vi "Autonomous Independent.vi"() -> ()   [LabVIEW 2016]
doc: "This VI is called when autonomous begins, and will automatically be terminated when autonomous ends. You can carry out timed or sensor driven robot movement independently without needing to return to the caller."
panel:
  out "ACTUAL Loop Time":u32
  # "Be sure to right-click and choose Data Operations>>Make Current Value default if you want to save the array values with the VI"
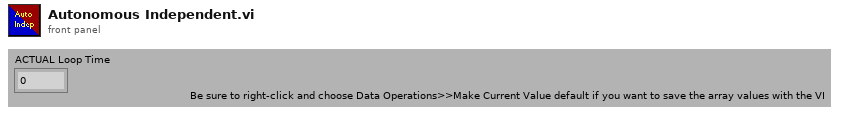
[diagram p1: front panel]
types:
  T1 = typedef "Autonomous Play Definition.ctl" = cluster{"Play Name":string, "Command List":cluster{"Param 1":dbl, "Param 2":dbl, "Autonomous Command Name":T2, "Concurrent":bool, "Param 3":dbl, "Param 4":string}[], "Play Description":string}
  T2 = typedef "Autonomous Command Names.ctl" = enum16{"No Op", "Command Drive+Climb Shift", "Command Wait", "Command Deliver Gear", "Command Buffer", "Command Drive Path", "Command Drive Time", "Command Shoot", "Command Turn to Heading", "Command Run Conveyor", "Command Spinup Shooter", "Command Deliver Gear Front", "Command Toggle Intake Rotation", "DO NOT USE", "Command Agitate Hopper", "Command Pre-Buffer", "Command Turn to Target", "Command Deliver Gear with Safety", "Command Drive Time with IMU", "Command Drive to Encoders"}
  T3 = typedef "All Robot Commands.ctl" = cluster{"Drive/Climb Commands":T4, "Gear Delivery Commands":T5, "Shooter and Conveyor Commands":T6, "Ball Intake Commands":T7}
  T4 = typedef "Drive + Climb Commands 2017.ctl" = cluster{"Robot Forward-Back":dbl, "Robot Twist":dbl, "High/Low Gear Shift":bool, "Toggle Left Climb Shifter":bool, "Toggle Right Climb Shifter":bool, "Enable Automatic Shifting":bool, "Enable Climb Motor ":bool}
  T5 = typedef "Gear Delivery Commands.ctl" = cluster{"Toggle Gear Release":bool, "Toggle Intake Rotation and Chute Door":bool, "Toggle Gear LED":bool}
  T6 = typedef "Conveyor and Shooter Commands.ctl" = cluster{"Toggle Shooter":bool, "Manual Reverse Conveyor":bool, "Run Feed System":bool, "Bump Down Flywheel Speed":bool, "Bump Up Flywheel Speed":bool}
  T7 = typedef "Ball Intake Commands.ctl" = cluster{"Toggle Ball Intake":bool, "Manual Reverse Intake":bool, "Toggle Ball Intake LED":bool}
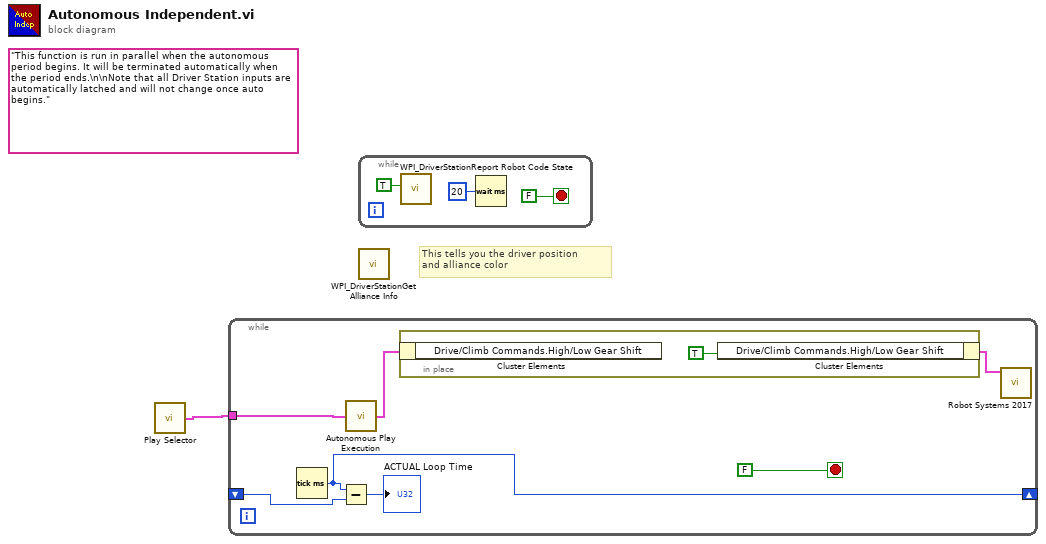
[diagram p0: block diagram]
diagram:
  (unwired) "This function is run in parallel when the autonomous period begins. It will be terminated automatically when the period ends.\n\nNote that all Driver Station inputs are automatically latched and will not change once auto begins."
  # "This tells you the driver position\nand alliance color"
  n1 = call "Play Selector.vi"() -> ("Output Play"=w1:T1)  [unwired: 1 in]
  n2 = while {
    shift-right: [w4] -> _
    shift-left: _ -> [w7]
    tunnel: w1 -> [w5]
    stop <- FALSE stop-if-true
    n3 = Tick Count (ms)() -> (millisecond timer value=w4:u32)
    n4 = Subtract(x=w4, y=w7) -> (x-y=→"ACTUAL Loop Time":u32)
    n5 = call "Autonomous Play Execution.vi"("Play 1"=w5) -> ("All Robot Commands Out"=w3:T3)
    n6 = in-place {
      n7 = in-place-cluster #1(w3) -> ()  [unwired: 1 out]
      n8 = in-place-cluster #1("Drive/Climb Commands.High/Low Gear Shift"=TRUE) -> (w2:T3)
    }
    n9 = call "Robot Systems 2017.vi"("All Robot Commands"=w2) -> ()  [unwired: 11 in]
  }
  n10 = while {
    stop <- FALSE stop-if-true
    n11 = call <vilib>:"WPI_DriverStationReport Robot Code State.vi"("Autonomous"=TRUE) -> ()  [unwired: 10 in, 1 out]
    n12 = Wait (ms)(milliseconds to wait=u32 20) -> ()  [unwired: 1 out]
  }
  n13 = call <vilib>:"WPI_DriverStationGet Alliance Info.vi"() -> ()  [unwired: 12 out]
